vi "SetROI.vi"(7 "Global Rectangle":i32[](array[numeric]), 9 "ROI In":T2, 10 "ROI Status":bool, 11 "Image In":T1) -> (1 "ROI Out":T2, 3 "Image Out":T1, 4 "y pixels":i32=512, 5 "xpixels":i32=512)   [LabVIEW 2015]
uses:
  <vilib>/vision/Image Controls.llb/IMAQ Image.ctl
  LiveImage_Global.vi
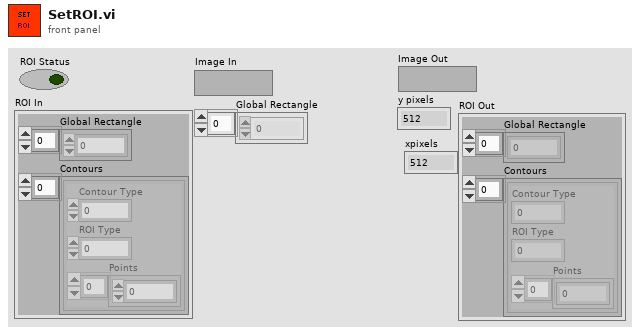
[diagram p1: front panel]
types:
  T1 = typedef "IMAQ Image.ctl" = refnum<image>
  T2 = cluster{"Global Rectangle":i32[], "Contours":cluster{"Contour Type":u32, "ROI Type":u32, "Points":i32[]}[]}
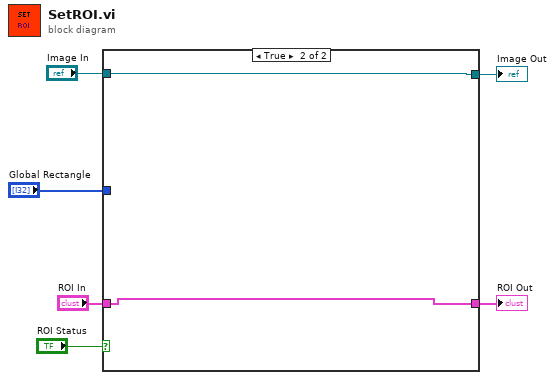
[diagram p0: block diagram]
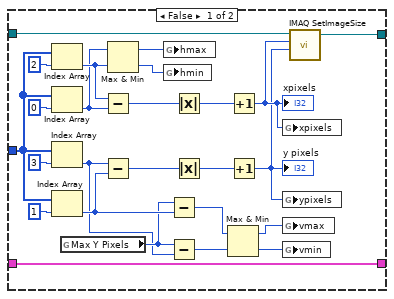
[diagram p2: hidden frame]
diagram:
  n1 = case shown="True" "ROI Status" {
    tunnel: "Global Rectangle" -> [w27 _]
    tunnel: "ROI In" -> [w16 w32]
    tunnel: [w16 w32] -> w4
    tunnel: "Image In" -> [w15 w33]
    tunnel: [w14 w33] -> w2
    frame False {
      n2 = Index Array(array=w27, index=2) -> (element=w26:i32)
      n3 = Index Array(array=w27, index=0) -> (element=w25:i32)
      n4 = Index Array(array=w27, index=3) -> (element=w8:i32)
      n5 = Index Array(array=w27, index=1) -> (element=w11:i32)
      n6 = global read "LiveImage_Global.vi" "Max Y Pixels"() -> (w9:i32)
      n7 = Subtract(x=w26, y=w25) -> (x-y=w24:i32)
      n8 = Subtract(x=w8, y=w11) -> (x-y=w23:i32)
      n9 = Max & Min(x=w25, y=w26) -> (max(x,y)=w20:i32, min(x,y)=w19:i32)
      n10 = global write "LiveImage_Global.vi" "hmax"(w20) -> ()
      n11 = global write "LiveImage_Global.vi" "hmin"(w19) -> ()
      n12 = Subtract(x=w9, y=w11) -> (x-y=w10:i32)
      n13 = Subtract(x=w9, y=w8) -> (x-y=w7:i32)
      n14 = Absolute Value(x=w24) -> (abs(x)=w22:i32)
      n15 = Absolute Value(x=w23) -> (abs(x)=w21:i32)
      n16 = Max & Min(x=w10, y=w7) -> (max(x,y)=w18:i32, min(x,y)=w17:i32)
      n17 = Increment(x=w22) -> (x+1=w13:i32)
      "xpixels" <- w13
      n18 = Increment(x=w21) -> (x+1=w12:i32)
      "y pixels" <- w12
      n19 = global write "LiveImage_Global.vi" "xpixels"(w13) -> ()
      n20 = global write "LiveImage_Global.vi" "ypixels"(w12) -> ()
      n21 = global write "LiveImage_Global.vi" "vmax"(w18) -> ()
      n22 = global write "LiveImage_Global.vi" "vmin"(w17) -> ()
      n23 = call "IMAQ SetImageSize"("Y Resolution"=w12, "X Resolution"=w13, "Image"=w15) -> ("Image Out"=w14:T1)  [unwired: 2 in, 1 out]
    }
    frame True {
    }
  }
  "ROI Out" <- w4
  "Image Out" <- w2
